vi "PIgetpos.vi"(7 "Numeric":i32, 8 "error in":errorcluster, 10 "Axes to query":string[](array[string]), 11 "System no.":i32=1 min=1 max=4 step=1) -> (0 "error out":errorcluster, 2 "position":dbl)   [LabVIEW 2012]
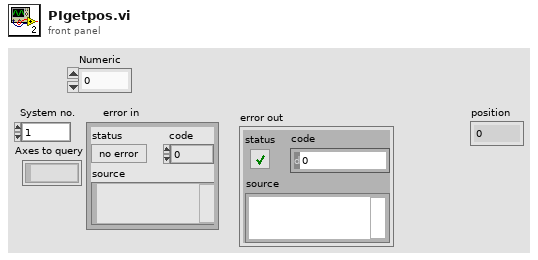
[diagram p1: front panel]
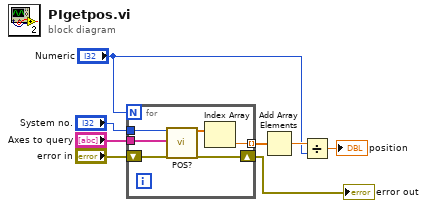
[diagram p0: block diagram]
diagram:
  n1 = for {
    N: "Numeric" -> [_]
    tunnel: "System no." -> [w14]
    tunnel: "Axes to query" -> [w13]
    tunnel: [w10] -> w5 mode=indexing
    shift-right: [w9] -> w1
    shift-left: "error in" -> [w12]
    n2 = call "POS?.vi"("System no."=w14, "Axes to query"=w13, "error in"=w12) -> ("Position"=w11:dbl[], "error out"=w9:errorcluster)  [unwired: 15 in]
    n3 = Index Array(array=w11) -> (element=w10:dbl)  [unwired: 1 in]
  }
  "error out" <- w1
  n4 = Add Array Elements(numeric array=w5) -> (sum=w4:dbl)
  n5 = Divide(x=w4, y="Numeric") -> (x/y=→"position":dbl)
